vi "DAQ6221 Thermocouples.vi"() -> ()   [LabVIEW 2020]
uses:
  <vilib>/DAQmx/read.llb/DAQmx Read (Analog 2D DBL NChan NSamp).vi
  <vilib>/Analysis/baseanly.llb/Mean (DBL).vi
  <vilib>/Utility/file.llb/Write To Spreadsheet File (string).vi
  <vilib>/DAQmx/create/channels.llb/DAQmx Create Channel (AI-Temperature-Thermocouple).vi
  <vilib>/DAQmx/configure/timing.llb/DAQmx Timing (Sample Clock).vi
  <vilib>/DAQmx/miscellaneous.llb/DAQmx Fill In Error Info.vi
  <vilib>/Utility/file.llb/Write To Spreadsheet File (DBL).vi
  <vilib>/Analysis/NI_AALBase.lvlib
panel:
  in  "stop":bool
  out "error out":errorcluster
  in  "samples":i32=500
  out "Temp 4":dbl format="%#_4g"
  out "Temp 3":dbl format="%#_4g"
  out "Temp 2":dbl format="%#_4g"
  out "Temp":dbl format="%#_4g"
  in  "title 4":string="Thermocouple 4"
  in  "title 3":string="Thermocouple 3"
  in  "title 2":string="Thermocouple 2"
  in  "title":string="Thermocouple 1"
  out "Waveform Chart":T1(graph)
  in  "rate":dbl=1000.0 format="%0.2f"
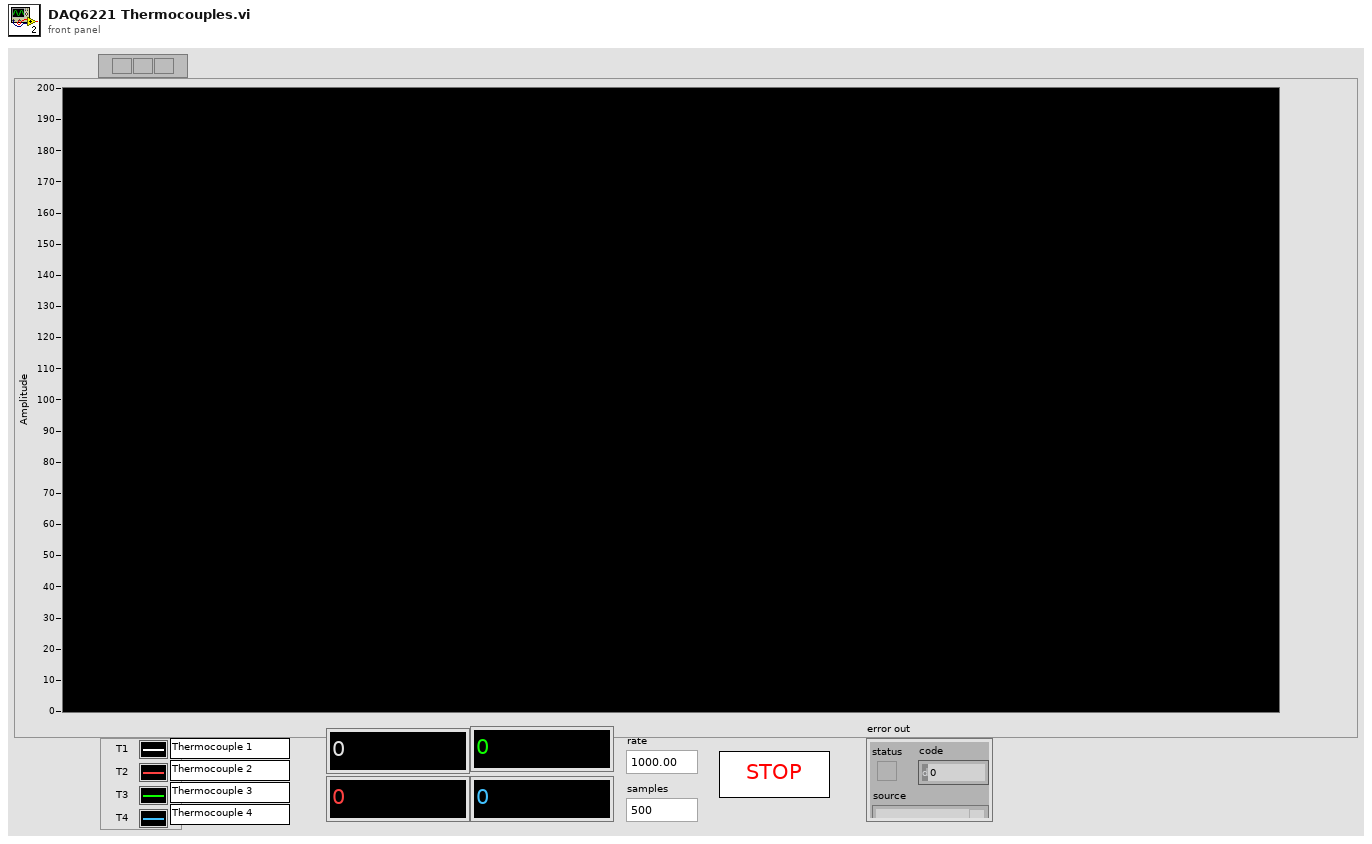
[diagram p1: front panel]
types:
  T1 = cluster{"mean":dbl, "mean":dbl, "mean":dbl, "mean":dbl}
  T2 = cluster{"mean":dbl, "mean":dbl, "mean":dbl, "mean":dbl}[]
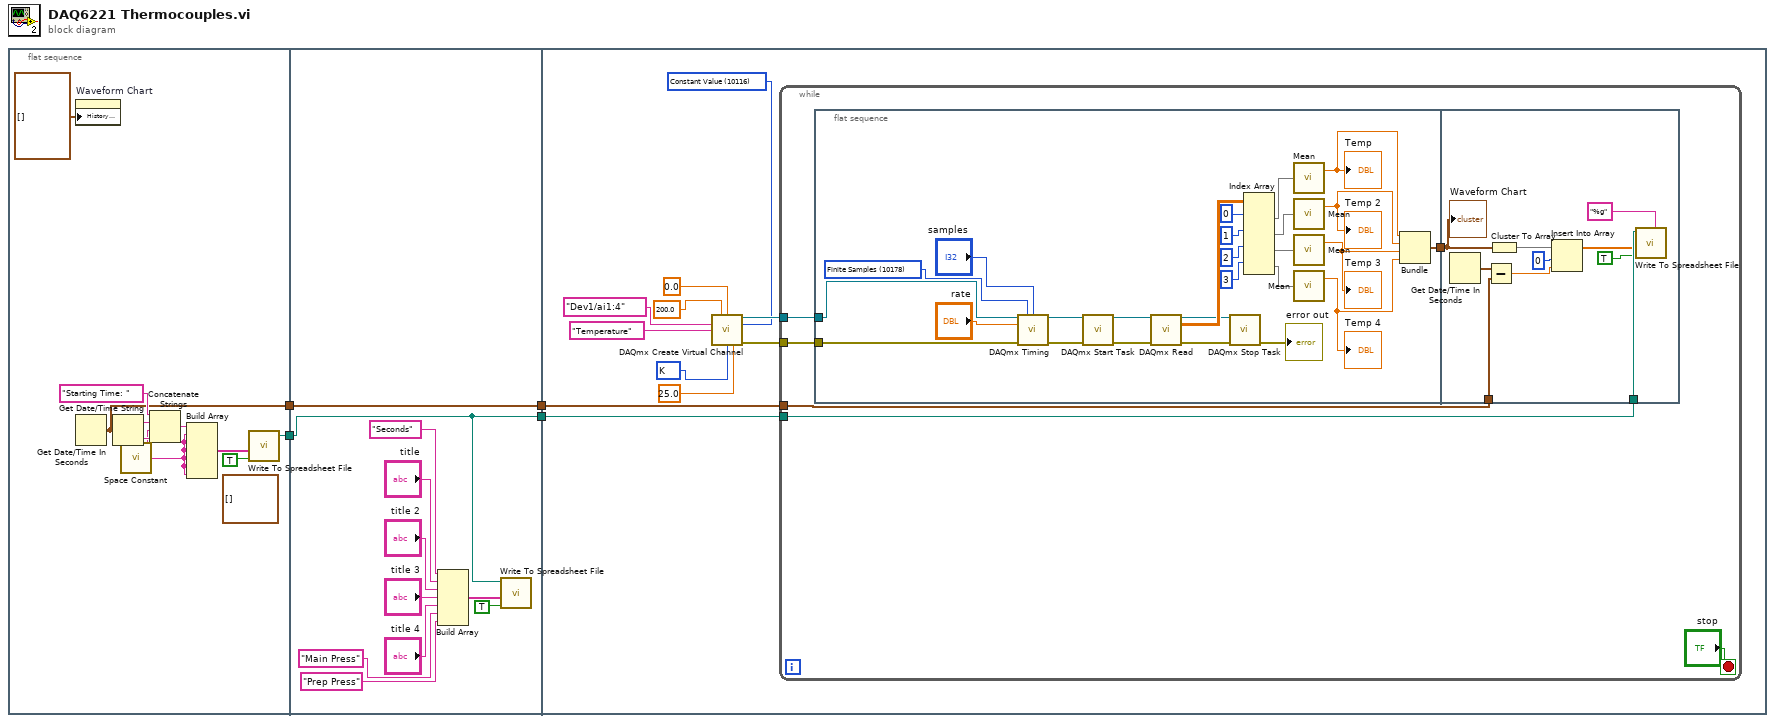
[diagram p0: block diagram]
diagram:
  n1 = flat-sequence {
    tunnel: [w13] -> w4
    tunnel: [w6] -> w1
    tunnel: w4 -> [w16]
    tunnel: [w16] -> w3
    tunnel: [w15] -> w2
    tunnel: w1 -> [w15]
    tunnel: w3 -> [w27]
    tunnel: w2 -> [w26]
    frame #0 {
      (unwired) cluster{"Output":dbl, "Output":dbl}[] [] ("History Data")
      n2 = property on="Waveform Chart" class="WFChart (strict)"("History Data"=T2 []) -> ()  [unwired: 2 in, 2 out]
      n3 = Get Date/Time In Seconds() -> (seconds since 1Jan1904=w6:timestamp)
      n4 = Get Date/Time String(seconds (now)=w6) -> (date string=w11:string, time string=w10:string)  [unwired: 2 in]
      n5 = call <vilib>:"Space Constant.vi"() -> ("String"=w8:string)
      n6 = Concatenate Strings("Starting Time: ", w11, w8, w10) -> (w9:string)
      n7 = Build Array(w9, w8, w8, w8, w8, w8, w8) -> (w7:string[])
      n8 = call-poly <vilib>:"Write To Spreadsheet File.vi"("append to file? (new file:F)"=TRUE, "1D data"=w7) -> ("new file path (Not A Path if cancelled)"=w13:path)  [unwired: 6 in]
    }
    frame #1 {
      n9 = Build Array("Seconds", "title", "title 2", "title 3", "title 4", "Main Press", "Prep Press") -> (w18:string[])
      n10 = call-poly <vilib>:"Write To Spreadsheet File.vi"("append to file? (new file:F)"=TRUE, "1D data"=w18, "file path (dialog if empty)"=w16) -> ()  [unwired: 5 in, 1 out]
    }
    frame #2 {
      w28 = 10116 items=["Built-In"=10200, "Constant Value"=10116, "Channel"=10113] ("cjc source")
      w35 = 10073 items=["J"=10072, "K"=10073, "N"=10077, "R"=10082, "S"=10085, "T"=10086, "B"=10047, "E"=10055] ("thermocouple type")
      n11 = call-poly <vilib>:"DAQmx Create Virtual Channel.vi"("maximum value"=200.0, "minimum value"=0.0, "physical channels"=tag "Dev1/ai1:4", "cjc source"=w28, "name to assign"="Temperature", "thermocouple type"=w35, "cjc value"=25.0) -> ("task out"=w30:refnum<k21>, "error out"=w29:errorcluster)  [unwired: 7 in]
      n12 = while {
        tunnel: w30 -> [w42]
        tunnel: w29 -> [w41]
        tunnel: w27 -> [w38]
        tunnel: w26 -> [w37]
        stop <- "stop" stop-if-true
        n13 = flat-sequence {
          tunnel: w42 -> [w68]
          tunnel: w41 -> [w67]
          tunnel: [w48] -> w39
          tunnel: w39 -> [w78]
          tunnel: w38 -> [w77]
          tunnel: w37 -> [w73]
          frame #0 {
            w66 = 10178 items=["Finite Samples"=10178, "Continuous Samples"=10123, "Hardware Timed Single Point"=12522] ("sample mode")
            n14 = call-poly <vilib>:"DAQmx Timing.vi"("task/channels in"=w68, "sample mode"=w66, "samples per channel"="samples", "rate"="rate", "error in"=w67) -> ("task out"=w63:refnum<k21>, "error out"=w62:errorcluster)  [unwired: 9 in]
            n15 = call <vilib>:"DAQmx Start Task.vi"("task/channels in"=w63, "error in"=w62) -> ("task out"=w61:refnum<k21>, "error out"=w60:errorcluster)  [unwired: 12 in]
            n16 = call-poly <vilib>:"DAQmx Read.vi"("task/channels in"=w61, "error in"=w60) -> ("task out"=w50:refnum<k21>, "data"=w59:dbl[][], "error out"=w49:errorcluster)  [unwired: 11 in]
            n17 = call <vilib>:"DAQmx Stop Task.vi"("task/channels in"=w50, "error in"=w49) -> ("error out"=→"error out":errorcluster)  [unwired: 12 in, 1 out]
            n18 = Index Array(array=w59, index (row) #1=0, index (row) #2=1, index (row) #3=2, index (row) #4=3) -> (element #1=w54:dbl[], element #2=w53:dbl[], element #3=w52:dbl[], element #4=w51:dbl[])  [unwired: 4 in]
            n19 = call-poly <vilib>:"Mean.vi"("X"=w54) -> ("mean"=w47:dbl)  [unwired: 1 out]
            "Temp" <- w47
            n20 = call-poly <vilib>:"Mean.vi"("X"=w53) -> ("mean"=w46:dbl)  [unwired: 1 out]
            "Temp 2" <- w46
            n21 = call-poly <vilib>:"Mean.vi"("X"=w52) -> ("mean"=w45:dbl)  [unwired: 1 out]
            "Temp 3" <- w45
            n22 = call-poly <vilib>:"Mean.vi"("X"=w51) -> ("mean"=w44:dbl)  [unwired: 1 out]
            "Temp 4" <- w44
            n23 = Bundle("mean"=w47, "mean"=w46, "mean"=w45, "mean"=w44) -> (w48:T1)  [unwired: 1 in]
          }
          frame #1 {
            n24 = Get Date/Time In Seconds() -> (seconds since 1Jan1904=w74:timestamp)
            n25 = Subtract(x=w74, y=w73) -> (x-y=w72:dbl)
            n26 = Cluster To Array(cluster=w78) -> (array=w69:dbl[])
            n27 = Insert Into Array(array=w69, index=0, new element=w72) -> (w70:dbl[])
            n28 = call-poly <vilib>:"Write To Spreadsheet File.vi"("format (%.3f)"="%g", "append to file? (new file:F)"=TRUE, "1D data"=w70, "file path (dialog if empty)"=w77) -> ()  [unwired: 4 in, 1 out]
            "Waveform Chart" <- w78
          }
        }
      }
    }
  }
